vi "macro_MecaDriveOdomNew.vi"   [LabVIEW 2019, in "Trajectory_Library.lvlib"]
uses:
  Trajectory_Library.lvlib
types:
  T1 = typedef "Trajectory_Library.lvlib/TRANSLATION2D.ctl" = cluster{"X":dbl, "Y":dbl}
  T2 = typedef "Trajectory_Library.lvlib/MECA_WHEEL_POSITIONS.ctl" = cluster{"FrontLeft":dbl, "FrontRight":dbl, "RearLeft":dbl, "RearRight":dbl, "P":bool}
  T3 = typedef "Trajectory_Library.lvlib/ROTATION2D.ctl" = cluster{"VALUE":dbl, "COS":dbl, "SIN":dbl}
  T4 = typedef "Trajectory_Library.lvlib/POSE2D.ctl" = cluster{"TRANSLATION":T1, "ROTATION":T3}
  T5 = typedef "Trajectory_Library.lvlib/MECA_DRIVE_KINEMATICS.ctl" = cluster{"FrontLeft":T1, "FrontRight":T1, "RearLeft":T1, "RearRight":T1, "InverseKinematics":T6, "ForwardKinematics":T6, "PrevCoR":T1}
  T6 = typedef "NI_Matrix.lvlib/RealMatrix.ctl" = dbl[][]
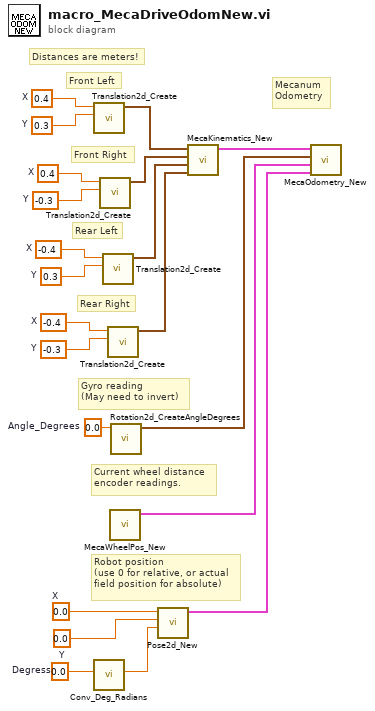
[diagram p0: block diagram]
diagram:
  w2 = 0.0  # Angle_Degrees
  w3 = 0.0  # Degress
  w4 = 0.0  # X
  w5 = 0.0  # Y
  w14 = -0.4  # X
  w15 = -0.3  # Y
  w16 = -0.4  # X
  w17 = 0.3  # Y
  w18 = 0.4  # X
  w19 = -0.3  # Y
  w20 = 0.4  # X
  w21 = 0.3  # Y
  # "Mecanum\nOdometry"
  # "Distances are meters!"
  # "Robot position\n(use 0 for relative, or actual \nfield position for absolute)"
  # "Current wheel distance\nencoder readings."
  # "Gyro reading\n(May need to invert)"
  # "Rear Right"
  # "Rear Left"
  # "Front Right"
  # "Front Left"
  n1 = call "Translation2d_Create.vi"("Y"=w21, "X"=w20) -> ("TRANSLATION"=w13:T1)  [unwired: 9 in]
  n2 = call "Conv_Deg_Radians.vi"("Degress"=w3) -> ("Radians"=w6:dbl)  [unwired: 10 in]
  n3 = call "Translation2d_Create.vi"("Y"=w19, "X"=w18) -> ("TRANSLATION"=w12:T1)  [unwired: 9 in]
  n4 = call "Translation2d_Create.vi"("Y"=w17, "X"=w16) -> ("TRANSLATION"=w11:T1)  [unwired: 9 in]
  n5 = call "Translation2d_Create.vi"("Y"=w15, "X"=w14) -> ("TRANSLATION"=w10:T1)  [unwired: 9 in]
  n6 = call "MecaWheelPos_New.vi"() -> ("MECA_WHEEL_POSITIONS"=w7:T2)  [unwired: 11 in]
  n7 = call "Rotation2d_CreateAngleDegrees.vi"("Angle_Degrees"=w2) -> ("ROTATION"=w8:T3)  [unwired: 10 in]
  n8 = call "Pose2d_New.vi"("Heading"=w6, "Y"=w5, "X"=w4) -> ("out POSe"=w1:T4)  [unwired: 8 in]
  n9 = call "MecaKinematics_New.vi"("RearRight"=w10, "RearLeft"=w11, "FrontRight"=w12, "FrontLeft"=w13) -> ("MECA_DRIVE_KINEMATICS"=w9:T5)  [unwired: 7 in]
  n10 = call "MecaOdometry_New.vi"("Initial Pose2d"=w1, "wheelPositions"=w7, "GyroOffset"=w8, "Mecanum Kinematics"=w9) -> ()  [unwired: 7 in, 1 out]
